vi "kDSA02.vi"(6 "max actuator":dbl, 8 "DSA Control Variables":T1={"High Freq"=200.0, "Sample Time"=0.001, "Low Freq"=10.0, "Num Data Points"=10, "Num Periods"=10, "Settling Time"=0.1}, 9 "min sens":dbl, 10 "max sens":dbl, 11 "Sensor Reading":dbl) -> (0 "Imag":dbl[](array[numeric]), 1 "Re":dbl[](array[numeric]), 2 "Frequencies":dbl[](array[numeric]), 3 "excitation signal":dbl)   [LabVIEW 2010, in "kevLib2011.lvlib"]
uses:
  kevLib2011.lvlib
  DSACntVariables.ctl
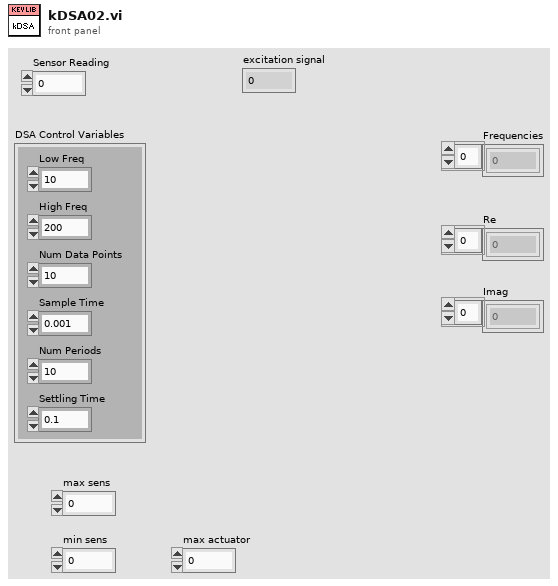
[diagram p1: front panel]
types:
  T1 = typedef "kevLib2011.lvlib/DSACntVariables.ctl" = cluster{"High Freq":dbl, "Sample Time":dbl, "Low Freq":dbl, "Num Data Points":i32, "Num Periods":i32, "Settling Time":dbl}
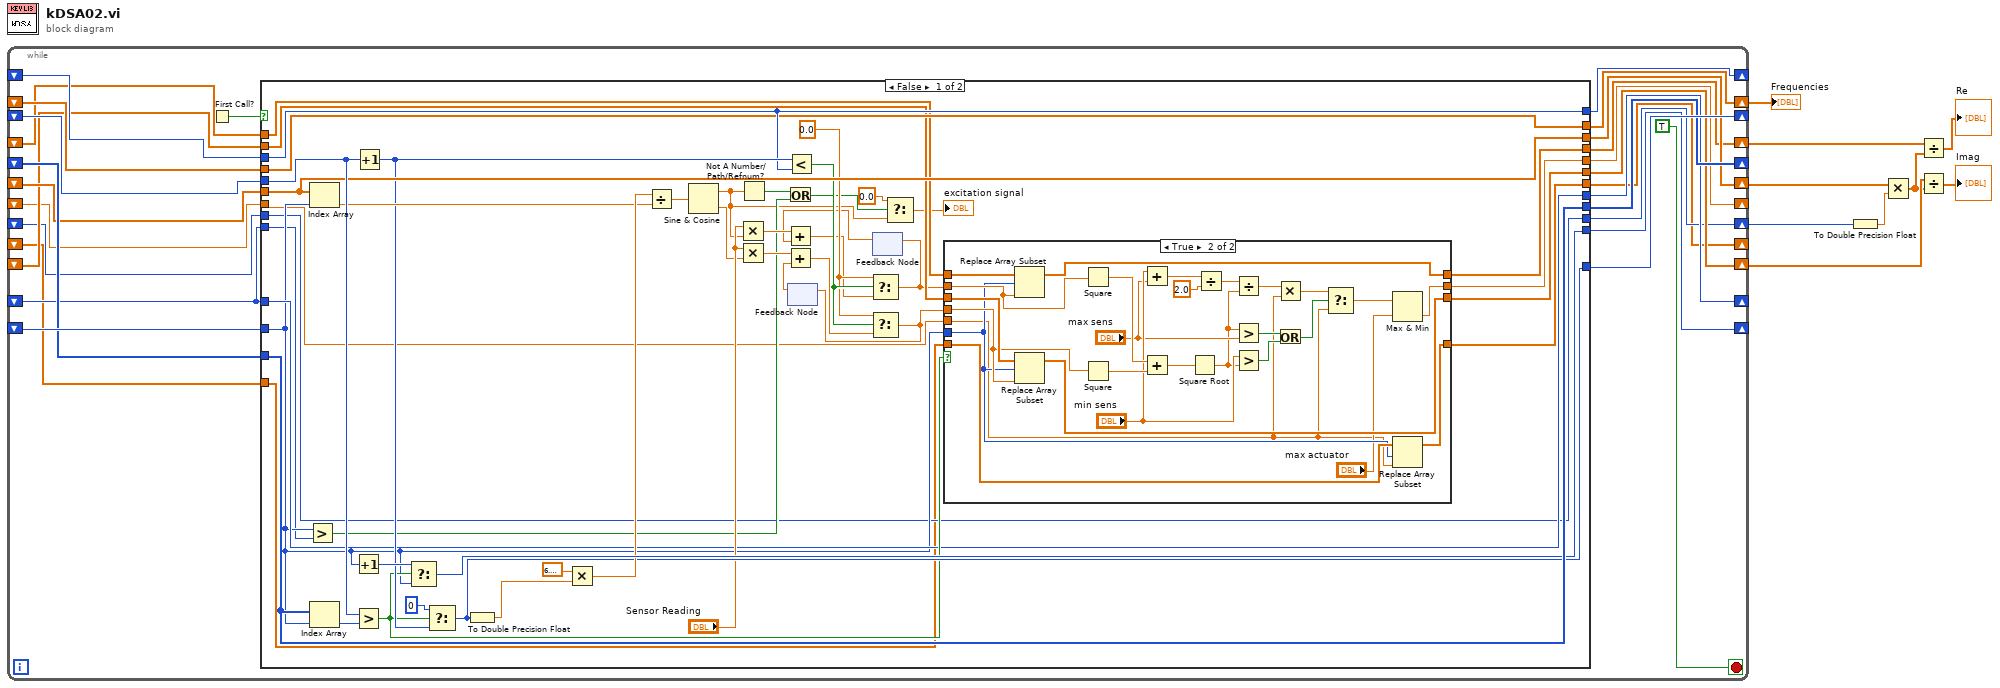
[diagram p0: block diagram]
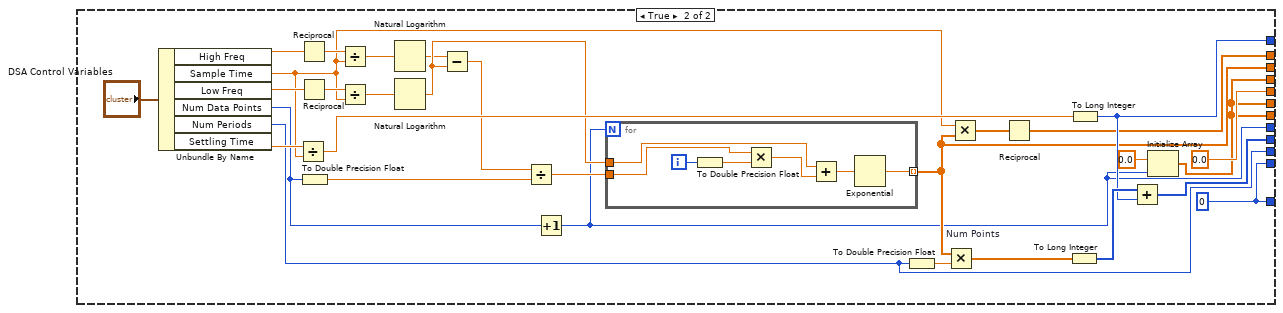
[diagram p3: hidden frame]
diagram:
  n1 = while {
    shift-right: [w33] -> _
    shift-left: _ -> [w32]
    shift-right: [w31] -> _
    shift-left: _ -> [w30]
    shift-right: [w29] -> _
    shift-left: _ -> [w28]
    shift-right: [w27] -> w2
    shift-left: _ -> [w26]
    shift-right: [w25] -> _
    shift-left: _ -> [w24]
    shift-right: [w21] -> w9
    shift-left: _ -> [w20]
    shift-right: [w23] -> w5
    shift-left: _ -> [w19]
    shift-right: [w22] -> w7
    shift-left: _ -> [w18]
    shift-right: [w17] -> _
    shift-left: _ -> [w16]
    shift-right: [w15] -> w3
    shift-left: _ -> [w14]
    shift-right: [w12] -> _
    shift-left: _ -> [w11]
    shift-right: [w13] -> _
    shift-left: _ -> [w10]
    stop <- TRUE stop-if-true
    n2 = First Call?() -> (First Call?: T/F=w34:bool)
    n3 = case shown="False" w34 {
      tunnel: [w72 w127] -> w33
      tunnel: w32 -> [w81 _]
      tunnel: [w77 w127] -> w31
      tunnel: w30 -> [w48 _]
      tunnel: [w80 w125] -> w29
      tunnel: w28 -> [w80 _]
      tunnel: [w71 w119] -> w27
      tunnel: w26 -> [w71 _]
      tunnel: [w64 w123] -> w25
      tunnel: w24 -> [w64 _]
      tunnel: [w52 w114] -> w23
      tunnel: [w51 w114] -> w22
      tunnel: [w57 w120] -> w21
      tunnel: w20 -> [w57 _]
      tunnel: w19 -> [w56 _]
      tunnel: w18 -> [w55 _]
      tunnel: [w49 w117] -> w17
      tunnel: w16 -> [w49 _]
      tunnel: w16 -> [w47 _]
      tunnel: [w40 w116] -> w15
      tunnel: w14 -> [w40 _]
      tunnel: [w36 0.0 ("element")] -> w13
      tunnel: [w38 w114] -> w12
      tunnel: w11 -> [w39 _]
      tunnel: w10 -> [w37 _]
      frame False {
        w62 = 0.0 ("t")
        n4 = Greater?(x=w48, y=w47) -> (0:w43:bool)
        n5 = Index Array(array=w71, index=w48) -> (element=w70:dbl)
        n6 = Index Array(array=w80, index=w48) -> (element=w79:i32)
        n7 = Increment(x=w48) -> (x+1=w78:i32)
        n8 = Greater?(x=w81, y=w79) -> (0:w50:bool)
        n9 = Increment(x=w81) -> (x+1=w65:i32)
        n10 = Select(t=w78, s=w50, f=w48) -> (s? t:f=w77:i32)
        n11 = Select(t=0, s=w50, f=w65) -> (s? t:f=w72:i32)
        n12 = To Double Precision Float(number=w72) -> (double precision float=w73:dbl)
        n13 = Multiply(x=6.283185307179586, y=w73) -> (x*y=w75:dbl)
        n14 = Divide(x=w75, y=w70) -> (x/y=w76:dbl)
        n15 = Sine & Cosine(0:w76) -> (1:w41:dbl, 2:w68:dbl)
        n16 = Multiply(x="Sensor Reading", y=w41) -> (x*y=w67:dbl)
        n17 = Multiply(x="Sensor Reading", y=w68) -> (x*y=w66:dbl)
        n18 = Not A Number/Path/Refnum?(number/path/refnum=w41) -> (NaN/Path/Refnum?=w44:bool)
        n19 = Or(x=w44, y=w43) -> (x .or. y?=w42:bool)
        n20 = Less?(x=w65, y=w64) -> (x < y?=w63:bool)
        n21 = feedback #1() -> (w59:dbl)  [unwired: 1 in]
        n22 = Add(x=w66, y=w59) -> (x+y=w58:dbl)
        n23 = Select(t=w62, s=w63, f=w58) -> (s? t:f=w53:dbl)
        n24 = feedback-in #1(w53) -> ()
        n25 = feedback #2() -> (w61:dbl)  [unwired: 1 in]
        n26 = Add(x=w67, y=w61) -> (x+y=w60:dbl)
        n27 = Select(t=w62, s=w63, f=w60) -> (s? t:f=w54:dbl)
        n28 = feedback-in #2(w54) -> ()
        n29 = Select(t=0.0, s=w42, f=w41) -> (s? t:f=→"excitation signal":dbl)
        n30 = case shown="True" w50 {
          tunnel: w56 -> [w86 w113]
          tunnel: w55 -> [w85 w112]
          tunnel: w48 -> [_ w91]
          tunnel: w54 -> [_ w109]
          tunnel: w53 -> [_ w108]
          tunnel: [w86 w111] -> w52
          tunnel: [w85 w110] -> w51
          tunnel: w39 -> [w84 w96]
          tunnel: [w84 w95] -> w38
          tunnel: w37 -> [w83 w87]
          tunnel: [w83 w88] -> w36
          frame False {
          }
          frame True {
            n31 = Replace Array Subset(array=w113, new element=w109, index=w91) -> (w111:dbl[])
            n32 = Replace Array Subset(array=w112, new element=w108, index=w91) -> (w110:dbl[])
            n33 = Square(x=w109) -> (x^2=w106:dbl)
            n34 = Square(x=w108) -> (x^2=w107:dbl)
            n35 = Add(x="min sens", y="max sens") -> (x+y=w100:dbl)
            n36 = Add(x=w106, y=w107) -> (x+y=w105:dbl)
            n37 = Square Root(x=w105) -> (sqrt(x)=w97:dbl)
            n38 = Divide(x=w100, y=2.0) -> (x/y=w98:dbl)
            n39 = Divide(x=w98, y=w97) -> (x/y=w92:dbl)
            n40 = Greater?(x=w97, y="max sens") -> (0:w104:bool)
            n41 = Greater?(x="min sens", y=w97) -> (0:w103:bool)
            n42 = Multiply(x=w92, y=w87) -> (x*y=w93:dbl)
            n43 = Or(x=w104, y=w103) -> (x .or. y?=w94:bool)
            n44 = Select(t=w93, s=w94, f=w87) -> (s? t:f=w90:dbl)
            n45 = Max & Min(x=w90, y="max actuator") -> (min(x,y)=w88:dbl)  [unwired: 1 out]
            n46 = Replace Array Subset(array=w96, new element=w87, index=w91) -> (w95:dbl[])
          }
        }
      }
      frame True {
        w127 = 0 ("32bit integer")
        n47 = Unbundle By Name("DSA Control Variables") -> ("High Freq"=w140:dbl, "Sample Time"=w121:dbl, "Low Freq"=w141:dbl, "Num Data Points"=w142:i32, "Num Periods"=w116:i32, "Settling Time"=w143:dbl)
        n48 = Divide(x=w143, y=w121) -> (x/y=w135:dbl)
        n49 = Reciprocal(x=w140) -> (1/x=w137:dbl)
        n50 = Reciprocal(x=w141) -> (1/x=w136:dbl)
        n51 = To Double Precision Float(number=w142) -> (double precision float=w130:dbl)
        n52 = Divide(x=w137, y=w121) -> (x/y=w134:dbl)
        n53 = Divide(x=w136, y=w121) -> (x/y=w133:dbl)
        n54 = Natural Logarithm(1:w134) -> (0:w128:dbl)
        n55 = Natural Logarithm(1:w133) -> (0:w132:dbl)
        n56 = Subtract(x=w128, y=w132) -> (x-y=w129:dbl)
        n57 = Divide(x=w129, y=w130) -> (x/y=w131:dbl)
        n58 = Increment(x=w142) -> (x+1=w117:i32)
        n59 = for {
          N: w117 -> [_]
          tunnel: w131 -> [w148]
          tunnel: w132 -> [w147]
          tunnel: [w144] -> w119 mode=indexing
          i -> [w150]
          n60 = To Double Precision Float(number=w150) -> (double precision float=w149:dbl)
          n61 = Multiply(x=w148, y=w149) -> (x*y=w146:dbl)
          n62 = Add(x=w147, y=w146) -> (x+y=w145:dbl)
          n63 = Exponential(1:w145) -> (0:w144:dbl)
        }
        n64 = To Double Precision Float(number=w116) -> (double precision float=w138:dbl)
        n65 = Multiply "Num Points"(x=w119, y=w138) -> (x*y=w124:dbl[])
        n66 = Multiply(x=w121, y=w119) -> (x*y=w122:dbl[])
        n67 = Reciprocal(x=w122) -> (1/x=w120:dbl[])
        n68 = To Long Integer(number=w124) -> (32bit integer=w126:i32[])
        n69 = To Long Integer(number=w135) -> (32bit integer=w123:i32)
        n70 = Add(x=w126, y=w123) -> (x+y=w125:i32[])
        n71 = Initialize Array(0.0 ("element"), w117) -> (w114:dbl[])
      }
    }
  }
  "Frequencies" <- w9
  n72 = To Double Precision Float(number=w3) -> (double precision float=w4:dbl)
  n73 = Multiply(x=w2, y=w4) -> (x*y=w1:dbl[])
  n74 = Divide(x=w5, y=w1) -> (x/y=→"Re":dbl[])
  n75 = Divide(x=w7, y=w1) -> (x/y=→"Imag":dbl[])
